vi "FuzzyTable.vi"(8 "Numeric":dbl) -> (0 "String":string)   [LabVIEW 2016]
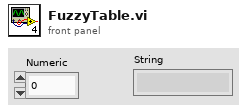
[diagram p1: front panel]
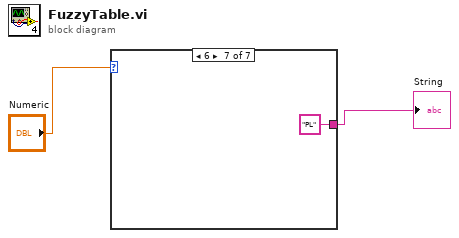
[diagram p0: block diagram]
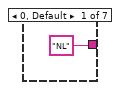
[diagram p2: hidden frame]
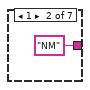
[diagram p3: hidden frame]
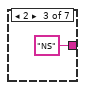
[diagram p4: hidden frame]
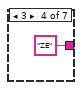
[diagram p5: hidden frame]
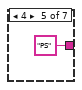
[diagram p6: hidden frame]
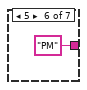
[diagram p7: hidden frame]
diagram:
  n1 = case shown="6" "Numeric" {
    tunnel: ["NL" ("String") "NM" ("String") "NS" ("String") "ZE" ("String") "PS" ("String") "PM" ("String") "PL" ("String")] -> w1
    frame 0, Default {
    }
    frame 1 {
    }
    frame 2 {
    }
    frame 3 {
    }
    frame 4 {
    }
    frame 5 {
    }
    frame 6 {
    }
  }
  "String" <- w1
